vi "Scale Data.vi"(8 "error in (no error)":errorcluster, 10 "Data":dbl[][](array[numeric]), 11 "VolatusScaling in":refnum<class "Scaling.lvclass">) -> (0 "error out":errorcluster, 2 "Scaled Data":dbl[][](array[numeric]))   [LabVIEW 2020, in "VolatusData.lvlib" / "Scaling.lvclass"]
uses:
  Scaling.lvclass
  Scaling.lvclass/Scaling.ctl
  Polynomial Remove Trailing Zeros.vi
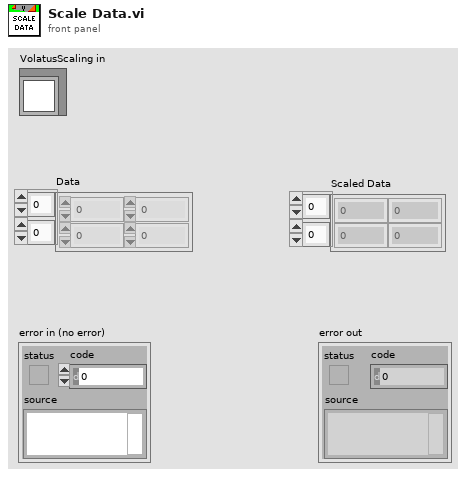
[diagram p1: front panel]
types:
  T1 = typedef "VolatusConfig.lvlib/Scale Type.ctl" = enum16{"None", "Sensor", "Polynomial", "Threshold", "Invert Bool"}
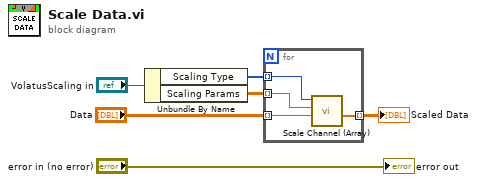
[diagram p0: block diagram]
diagram:
  n1 = Unbundle By Name("VolatusScaling in") -> ("Scaling Type"=w3:T1[], "Scaling Params"=w2:dbl[][])
  n2 = for {
    tunnel: "Data" -> [w10] mode=indexing
    tunnel: w3 -> [w8] mode=indexing
    tunnel: w2 -> [w9] mode=indexing
    tunnel: [w7] -> w1 mode=indexing
    n3 = call "Scale Channel (Array).vi"("Data"=w10, "Scaling Params"=w9, "Scaling Type"=w8) -> ("Scaled Data"=w7:dbl[])  [unwired: 8 in]
  }
  "Scaled Data" <- w1
  "error out" <- "error in (no error)"
